vi "Close Door.vi"(8 "error in (no error)":errorcluster, 11 "Doors Opening in":refnum<class "Doors Opening.lvclass">) -> (0 "error out":errorcluster, 3 "Doors Opening out":refnum<class "Doors Opening.lvclass">)   [LabVIEW 2020, in "Door Controller.lvlib" / "Doors Opening.lvclass"]
uses:
  Doors Opening.lvclass
  C:/Users/Thomas.McQuillan/Desktop/Elevator Door Control/Door Controller/Door Controller/Door Controller.lvclass
  Door Controller/Door Controller.lvclass/Door Controller.ctl
  <vilib>/ActorFramework/Message Enqueuer/Message Enqueuer.lvclass/Message Enqueuer.ctl
  <vilib>/ActorFramework/Message Enqueuer/Enqueue.vi
  Door Hardware/Door Hardware Messages/Close Doors Msg/Close Doors Msg.lvclass
  C:/Program Files/National Instruments/LabVIEW 2020/vi.lib/ActorFramework/Message/Message.lvclass
  <vilib>/ActorFramework/Message Priority Queue/Priority Enqueue.vi
  Door Controller/Door Controller.lvclass
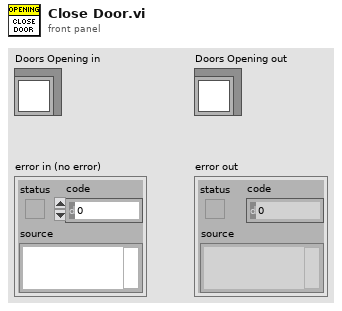
[diagram p1: front panel]
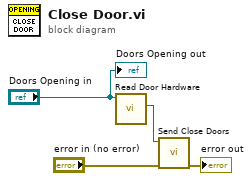
[diagram p0: block diagram]
diagram:
  n1 = call "Read Door Hardware.vi"("Door Controller in"="Doors Opening in") -> ("Door Hardware"=w3:refnum<class "Message Enqueuer.lvclass">)  [unwired: 10 in]
  n2 = call "Send Close Doors.vi"("error in (no error)"="error in (no error)", "Message Enqueuer"=w3) -> ("error out"=→"error out":errorcluster)  [unwired: 8 in, 1 out]
  "Doors Opening out" <- "Doors Opening in"
